vi "4 Comparison.vi"() -> ()   [LabVIEW 2015]
panel:
  out "EXCESSIVE":bool
  out "SAFE":bool
  out "Thermometer":dbl(slide) scale=0.0..100.0
  in  "Set Point":dbl
  in  "Temperature Sensor":dbl(knob) scale=0.0..100.0
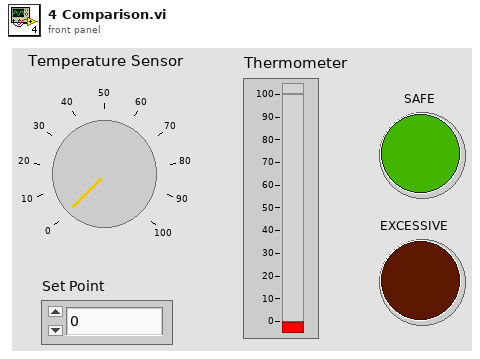
[diagram p1: front panel]
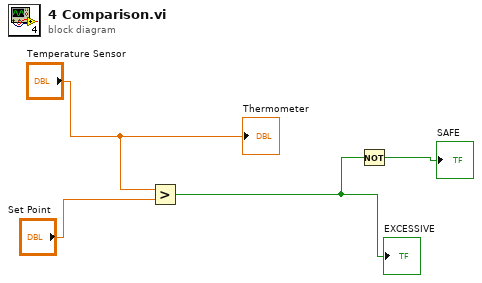
[diagram p0: block diagram]
diagram:
  n1 = Greater?(x="Temperature Sensor", y="Set Point") -> (0:w2:bool)
  "EXCESSIVE" <- w2
  n2 = Not(x=w2) -> (.not. x?=→"SAFE":bool)
  "Thermometer" <- "Temperature Sensor"
